vi "Determine Installed Modules.vi"(8 "error in":errorcluster, 11 "34980A in":refnum<class "34980A.lvclass">) -> (0 "error out":errorcluster, 3 "34980A out":refnum<class "34980A.lvclass">)   [LabVIEW 2019, in "34980A.lvlib" / "34980A.lvclass"]
uses:
  Library/34980A.lvclass
  Library/34980A.lvclass/34980A.ctl
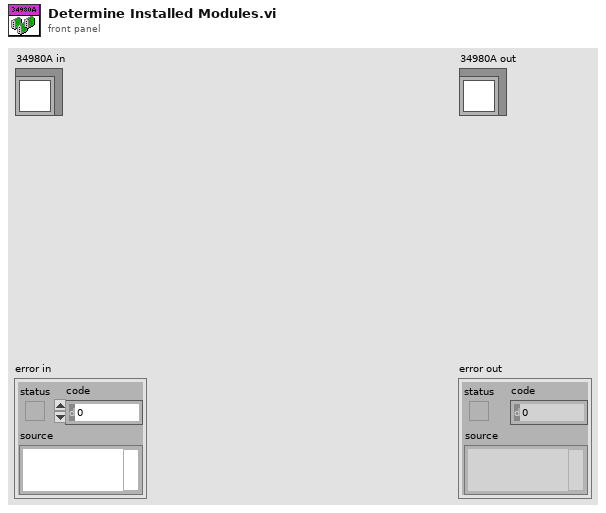
[diagram p1: front panel]
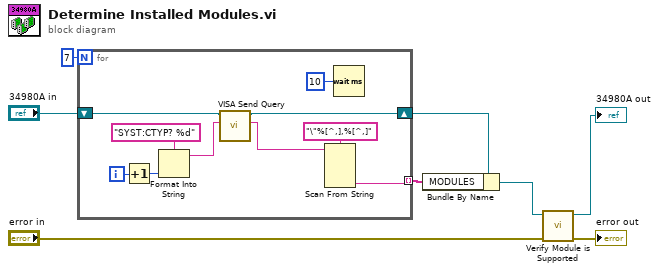
[diagram p0: block diagram]
diagram:
  n1 = for {
    N: 7 -> [_]
    shift-right: [w17] -> w6
    shift-left: "34980A in" -> [w18]
    tunnel: [w14] -> w5 mode=indexing
    i -> [w12]
    n2 = Increment(x=w12) -> (x+1=w13:i32)
    n3 = Format Into String(format string="SYST:CTYP? %d", w13) -> (resulting string=w10:string)  [unwired: 2 in, 1 out]
    n4 = call "VISA Send Query.vi"("Query"=w10, "34980A in"=w18) -> ("read buffer"=w15:string, "34980A out"=w17:refnum<class "34980A.lvclass">)  [unwired: 7 in, 1 out]
    n5 = Scan From String(format string="\"%[^,],%[^,]", input string=w15) -> (output 2=w14:string)  [unwired: 5 in, 3 out]
    n6 = Wait (ms)(milliseconds to wait=u32 10) -> ()  [unwired: 1 out]
  }
  n7 = Bundle By Name(cluster=w6, "MODULES"=w5) -> (w4:refnum<class "34980A.lvclass">)
  n8 = call "Verify Module is Supported.vi"("error in"="error in", "34980A in"=w4) -> ("error out"=→"error out":errorcluster, "34980A out"=→"34980A out":refnum<class "34980A.lvclass">)  [unwired: 8 in]
